vi "Log Error.vi"(6 "Clear error (T)":bool=TRUE, 8 "error in (no error)":errorcluster, 9 "Source":string, 11 "file path (use dialog)":path) -> (0 "error out":errorcluster)   [LabVIEW 2021]
doc: "Saves Error in Log file\nmay clear the error cluster"
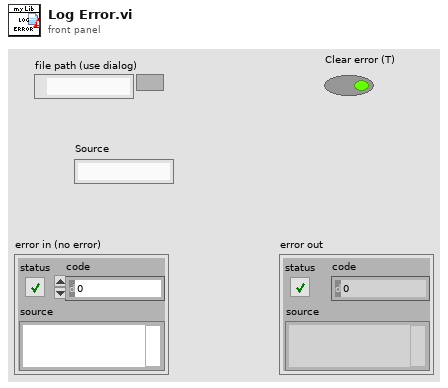
[diagram p1: front panel]
types:
  T1 = enum16{"open", "replace", "create", "open or create", "replace or create", "replace or create with confirmation"}
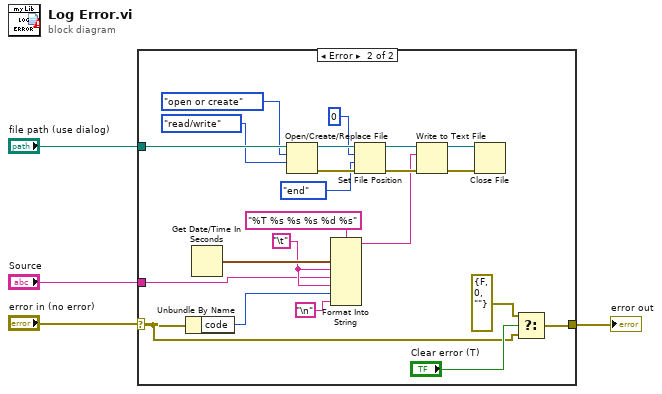
[diagram p0: block diagram]
diagram:
  n1 = case shown="Error" "error in (no error)" {
    selector: "error in (no error)" -> [w5 w10]
    tunnel: [w5 w12] -> w3
    tunnel: "file path (use dialog)" -> [_ w27]
    tunnel: "Source" -> [_ w8]
    frame No Error {
    }
    frame Error {
      w15 = "\t"
      n2 = Unbundle By Name(w10) -> ("code"=w14:i32)
      n3 = Get Date/Time In Seconds() -> (seconds since 1Jan1904=w16:timestamp)
      n4 = Open/Create/Replace File(file path (use dialog)=w27, operation (0:open)=T1."open or create", access (0:read/write)=enum16{"read/write", "read-only", "write-only"}."read/write") -> (refnum out=w24:refnum<file>, error out=w23:errorcluster)  [unwired: 3 in, 1 out]
      n5 = Format Into String(format string="%T %s %s %s %d %s", w16, w15, w8, w15, w14, "\n") -> (resulting string=w7:string)  [unwired: 2 in, 1 out]
      n6 = Set File Position(offset (in bytes) (0)=i64 0, refnum=w24, from (0:start)=enum16{"start", "end", "current"}."end", error in=w23) -> (refnum out=w20:refnum<file>, error out=w19:errorcluster)
      n7 = Write to Text File(file (use dialog)=w20, text=w7, error in=w19) -> (refnum out=w17:refnum<file>, error out=w18:errorcluster)  [unwired: 1 in, 1 out]
      n8 = Close File(refnum=w17, error in=w18) -> ()  [unwired: 2 out]
      n9 = Select(t=errorcluster {"status"=FALSE, "code"=0, "source"=""}, s="Clear error (T)", f=w10) -> (s? t:f=w12:errorcluster)
    }
  }
  "error out" <- w3
